vi "demux.vi"(4 "array":dbl[](array[numeric])) -> (0 "2":dbl, 1 "1":dbl, 2 "0":dbl)   [LabVIEW 2018]
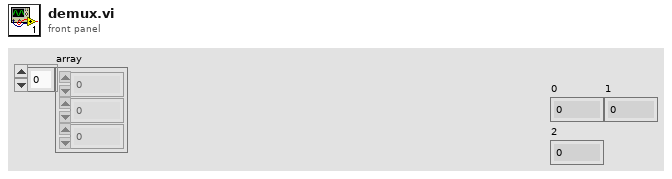
[diagram p1: front panel]
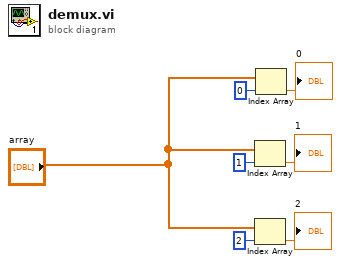
[diagram p0: block diagram]
diagram:
  n1 = Index Array(array="array", index=1) -> (element=→"1":dbl)
  n2 = Index Array(array="array", index=2) -> (element=→"2":dbl)
  n3 = Index Array(array="array", index=0) -> (element=→"0":dbl)
